vi "时间校准.vi"() -> (2 "DTout":u16[](array[numeric]) format="%x")   [LabVIEW 2020]
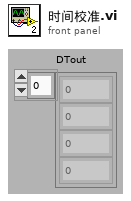
[diagram p1: front panel]
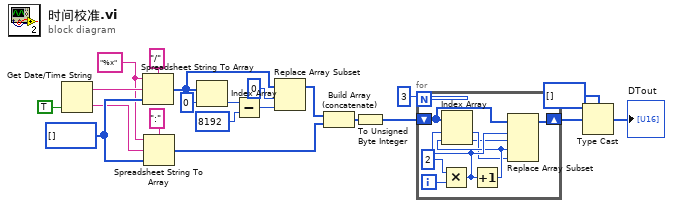
[diagram p0: block diagram]
diagram:
  w18 = "%x" ("格式字符串")
  w20 = u16[] [] ("数组类型(2D Dbl)")
  n1 = Get Date/Time String(want seconds? (F)=TRUE ("需要秒？(F)")) -> (date string=w21:string, time string=w19:string)  [unwired: 2 in]
  n2 = Spreadsheet String To Array(delimiter (Tab)="/" ("分隔符(Tab)"), format string=w18, spreadsheet string=w21, array type (2D Dbl)=w20) -> (array=w10:u16[])
  n3 = Spreadsheet String To Array(delimiter (Tab)=":" ("分隔符(Tab)"), format string=w18, spreadsheet string=w19, array type (2D Dbl)=w20) -> (array=w8:u16[])
  n4 = Index Array(array=w10, index=0 ("索引")) -> (element=w14:u16)
  n5 = Subtract(x=w14, y=u16 8192) -> (x-y=w12:u16)
  n6 = Replace Array Subset(array=w10, new element=w12, index=0 ("索引")) -> (w9:u16[])
  n7 = Build Array (concatenate)(w9, w8) -> (w7:u16[])
  n8 = To Unsigned Byte Integer(number=w7) -> (unsigned 8bit integer=w2:u8[])
  n9 = for {
    N: 3 -> [_]
    shift-right: [w22] -> w1
    shift-left: w2 -> [w27]
    i -> [w29]
    n10 = Multiply(x=2, y=w29) -> (x*y=w26:i32)
    n11 = Increment(x=w26) -> (x+1=w25:i32)
    n12 = Index Array(array=w27, index #1=w26, index #2=w25) -> (element #1=w24:u8, element #2=w23:u8)
    n13 = Replace Array Subset(array=w27, new element #1=w23, index #1=w26, new element #2=w24, index #2=w25) -> (w22:u8[])
  }
  n14 = Type Cast(type=u16[] [] ("Input Registers"), x=w1) -> (*(type *) &x=→"DTout":u16[])
